vi "REPORT XLS PEDROLLO.vi"(8 "template (empty)":path, 10 "Codice":string, 11 "report file path":path) -> ()   [LabVIEW 2016]
uses:
  <vilib>/Utility/NIReport.llb/NI_report.lvclass
  <vilib>/addons/_office/NI_ReportGenerationToolkit.lvlib
  <vilib>/Utility/NIReport.llb/Excel/NI_Excel.lvclass
  <vilib>/addons/database/NI_Database_API.lvlib
  <vilib>/addons/database/_DB Variant To Data/Database Variant To Data.xnode
  <vilib>/addons/_office/excel.llb/Excel Easy Table (str).vi
  <vilib>/Utility/NIReport.llb/Append Image to Report (path wrap).vi
  <vilib>/Utility/file.llb/Read Delimited Spreadsheet (string).vi
panel:
  out "P2":dbl
  out "toll REND":dbl
  out "toll P":dbl
  out "toll H":dbl
  out "toll Q":dbl
  out "H2":dbl
  out "H1":dbl
  out "Q2":dbl
  out "Q1":dbl
  in  "template (empty) 2":path
  in  "REPORT EXCEL":bool
  out "Nomi colonne":string[](array[string])
  in  "GRAFICA":bool
  in  "exit":bool
  in  "Interpola QP2":cluster{"interpola?":bool, "order":dbl}[](array[cluster])=[{"interpola?"=FALSE, "order"=2.0}, {"interpola?"=FALSE, "order"=2.0}, {"interpola?"=FALSE, "order"=2.0}, {"interpola?"=FALSE, "order"=2.0}, {"interpola?"=FALSE, "order"=2.0}, {"interpola?"=FALSE, "order"=2.0}, {"interpola?"=FALSE, "order"=2.0}, {"interpola?"=FALSE, "order"=2.0}, {"interpola?"=FALSE, "order"=2.0}, {"interpola?"=FALSE, "order"=2.0}, {"interpola?"=FALSE, "order"=2.0}, {"interpola?"=FALSE, "order"=2.0}, {"interpola?"=FALSE, "order"=2.0}, {"interpola?"=FALSE, "order"=2.0}, {"interpola?"=FALSE, "order"=2.0}, {"interpola?"=FALSE, "order"=2.0}, {"interpola?"=FALSE, "order"=2.0}, {"interpola?"=FALSE, "order"=2.0}] caption="Interpola?"
  in  "Interpola QRpm":cluster{"interpola?":bool, "order":dbl}[](array[cluster])=[{"interpola?"=FALSE, "order"=2.0}, {"interpola?"=FALSE, "order"=2.0}, {"interpola?"=FALSE, "order"=2.0}, {"interpola?"=FALSE, "order"=2.0}, {"interpola?"=FALSE, "order"=2.0}, {"interpola?"=FALSE, "order"=2.0}, {"interpola?"=FALSE, "order"=2.0}, {"interpola?"=FALSE, "order"=2.0}, {"interpola?"=FALSE, "order"=2.0}, {"interpola?"=FALSE, "order"=2.0}, {"interpola?"=FALSE, "order"=2.0}, {"interpola?"=FALSE, "order"=2.0}, {"interpola?"=FALSE, "order"=2.0}, {"interpola?"=FALSE, "order"=2.0}, {"interpola?"=FALSE, "order"=2.0}, {"interpola?"=FALSE, "order"=2.0}, {"interpola?"=FALSE, "order"=2.0}, {"interpola?"=FALSE, "order"=2.0}] caption="Interpola?"
  in  "Interpola QH":cluster{"interpola?":bool, "order":dbl}[](array[cluster])=[{"interpola?"=FALSE, "order"=2.0}, {"interpola?"=FALSE, "order"=2.0}, {"interpola?"=FALSE, "order"=2.0}, {"interpola?"=FALSE, "order"=2.0}, {"interpola?"=FALSE, "order"=2.0}, {"interpola?"=FALSE, "order"=2.0}, {"interpola?"=FALSE, "order"=2.0}, {"interpola?"=FALSE, "order"=2.0}, {"interpola?"=FALSE, "order"=2.0}, {"interpola?"=FALSE, "order"=2.0}, {"interpola?"=FALSE, "order"=2.0}, {"interpola?"=FALSE, "order"=2.0}, {"interpola?"=FALSE, "order"=2.0}, {"interpola?"=FALSE, "order"=2.0}, {"interpola?"=FALSE, "order"=2.0}, {"interpola?"=FALSE, "order"=2.0}, {"interpola?"=FALSE, "order"=2.0}, {"interpola?"=FALSE, "order"=2.0}] caption="Interpola?"
  in  "collaudi di confronto":string[](array[string])
  in  "carica collaudi di confronto":bool
  in  "Tab Control":T1(tab)
  in  "TABELLA 3":i32(listbox)
  in  "TABELLA 2":i32(listbox)
  in  "TABELLA 1":i32(listbox)
  in  "PLOT LEGEND QH-QP2":T2(array[cluster])
  in  "PLOT LEGEND QH-QRPM":T2(array[cluster])
  out "ProvaQH-QP2":cluster{"X":dbl[], "Y":dbl[]}[](graph)
  out "ProvaQH-QRpm":cluster{"X":dbl[], "Y":dbl[]}[](graph)
  out "ProvaQH-QH":cluster{"X":dbl[], "Y":dbl[]}[](graph)
  in  "PLOT LEGEND QH-QH":T2(array[cluster])
  in  "carica collaudo in corso":bool
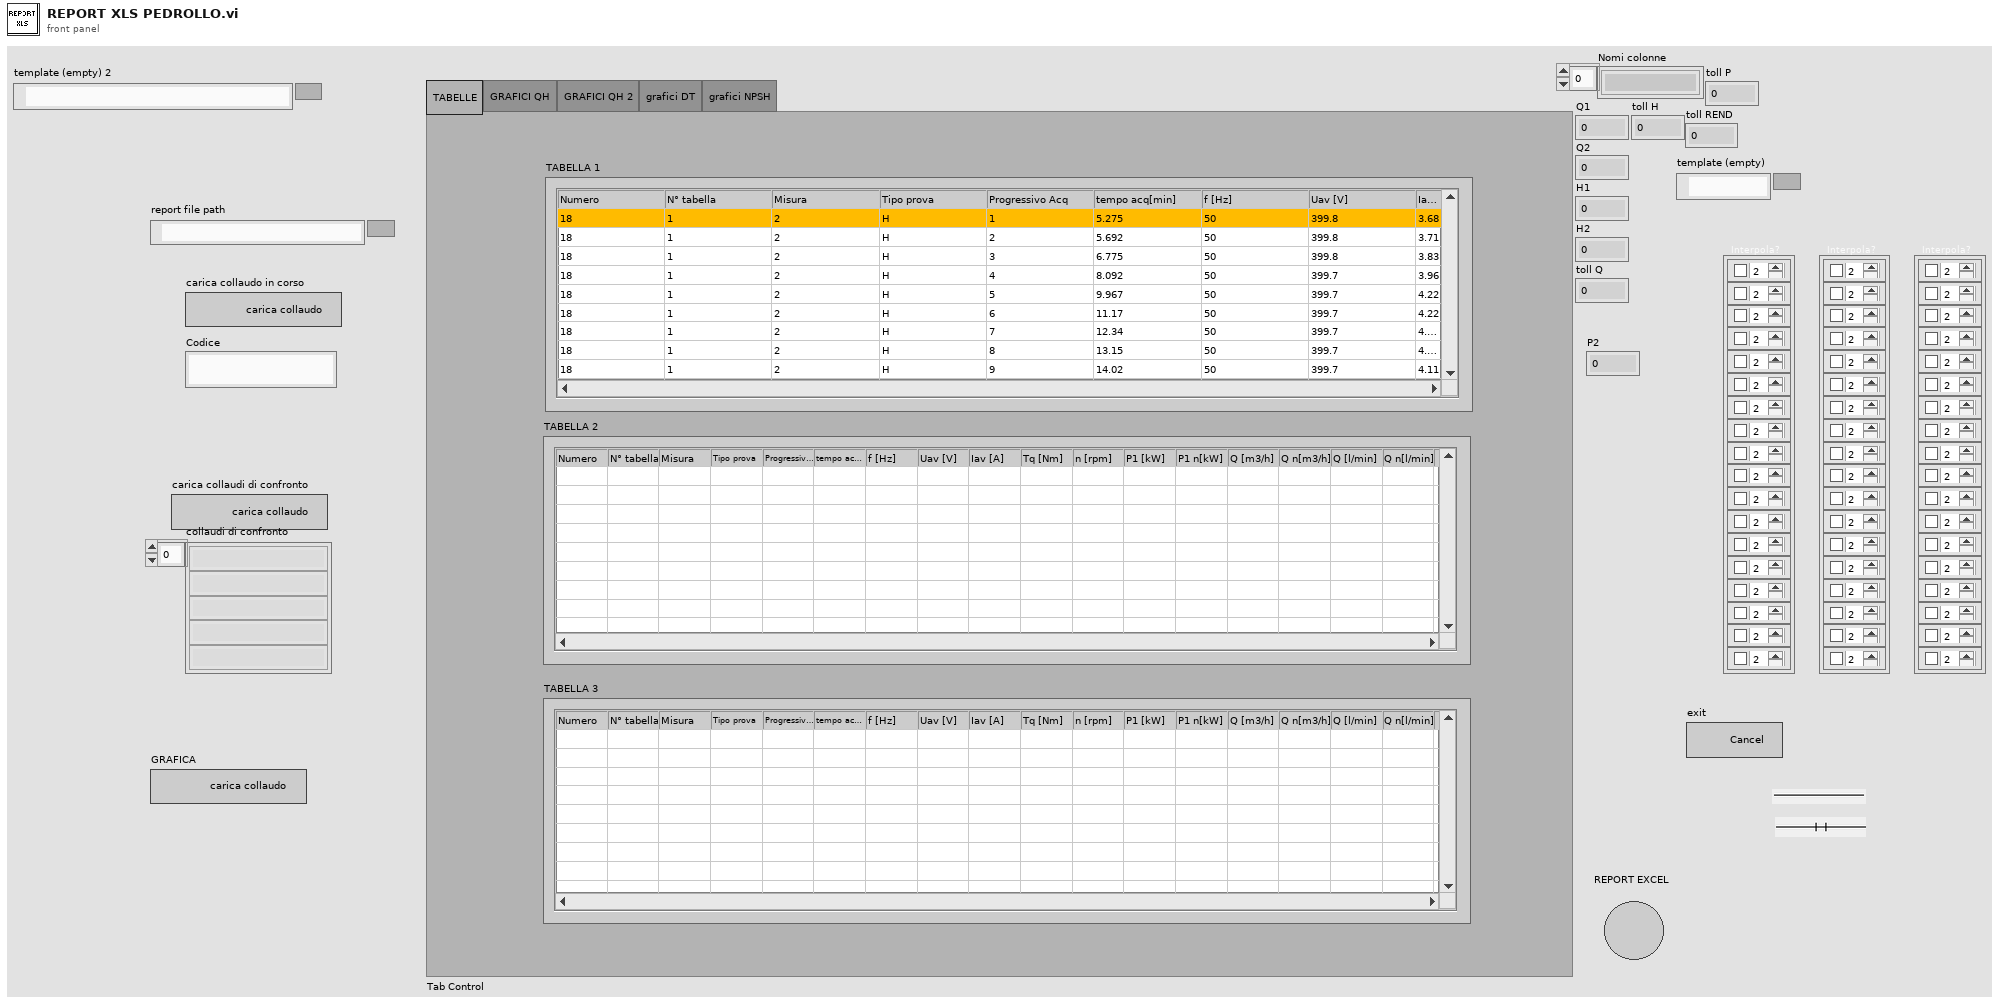
[diagram p1: front panel]
types:
  T1 = enum32{"TABELLE", "GRAFICI QH", "GRAFICI QH 2", "grafici DT", "grafici NPSH"}
  T2 = cluster{"nome plot":string, "colore":u32, "Larghezza linea":u16, "stile linea":u16, "stile punto":u16, "Visibile?":bool, "interpola?":bool, "ordine":dbl}[]
  T3 = cluster{"QH":cluster{"X":dbl[], "Y":dbl[]}[], "QRPM":cluster{"X":dbl[], "Y":dbl[]}[], "QP2":cluster{"X":dbl[], "Y":dbl[]}[]}
  T4 = enum16{"maximized", "minimized", "normal", "no change"}
  T5 = enum16{"Standard Report", "HTML", "Word", "Excel"}
  T6 = typedef "Indici.ctl" = cluster{"Q":i32, "Htot":i32, "NPSH":i32, "P3":i32, "etap":i32, "temperature":cluster{"DT":i32, "DTmarcia":i32, "DTaux":i32, "TC1":i32, "TC2":i32, "TC3":i32, "TC4":i32}, "tempo":i32, "P2":i32, "P1":i32, "etaGr":i32, "RPM":i32}
  T7 = cluster{"position (Excel)":cluster{"row":i32, "column":i32}, "name (Excel)":string, "bookmark (Word)":string}
  T8 = typedef "NI_Database_API.lvlib/Conn ObjectReference.ctl" = refnum<k1>
  T9 = typedef "Dati collaudo.ctl" = cluster{"QH freddo":T10, "QH regime":T10, "DT":T10, "NPSH":T10, "MEI":T10, "nome collaudo":string, "ResFreddo":cluster{"Curva 1":string[][]}}
  T10 = typedef "Curve prova.ctl" = cluster{"Curva 1":string[][], "Curva 2":string[][], "Curva 3":string[][]}
  T11 = cluster{"nome plot":string, "colore":u32, "Larghezza linea":u16, "stile linea":u16, "stile punto":u16, "Visibile?":bool, "interpola?":bool, "ordine":dbl}
  T12 = typedef "imagedata.ctl" = cluster{"image type":i32, "image depth":i32, "image":u8[], "mask":u8[], "colors":u32[], "Rectangle":cluster{"left":i16, "top":i16, "right":i16, "bottom":i16}}
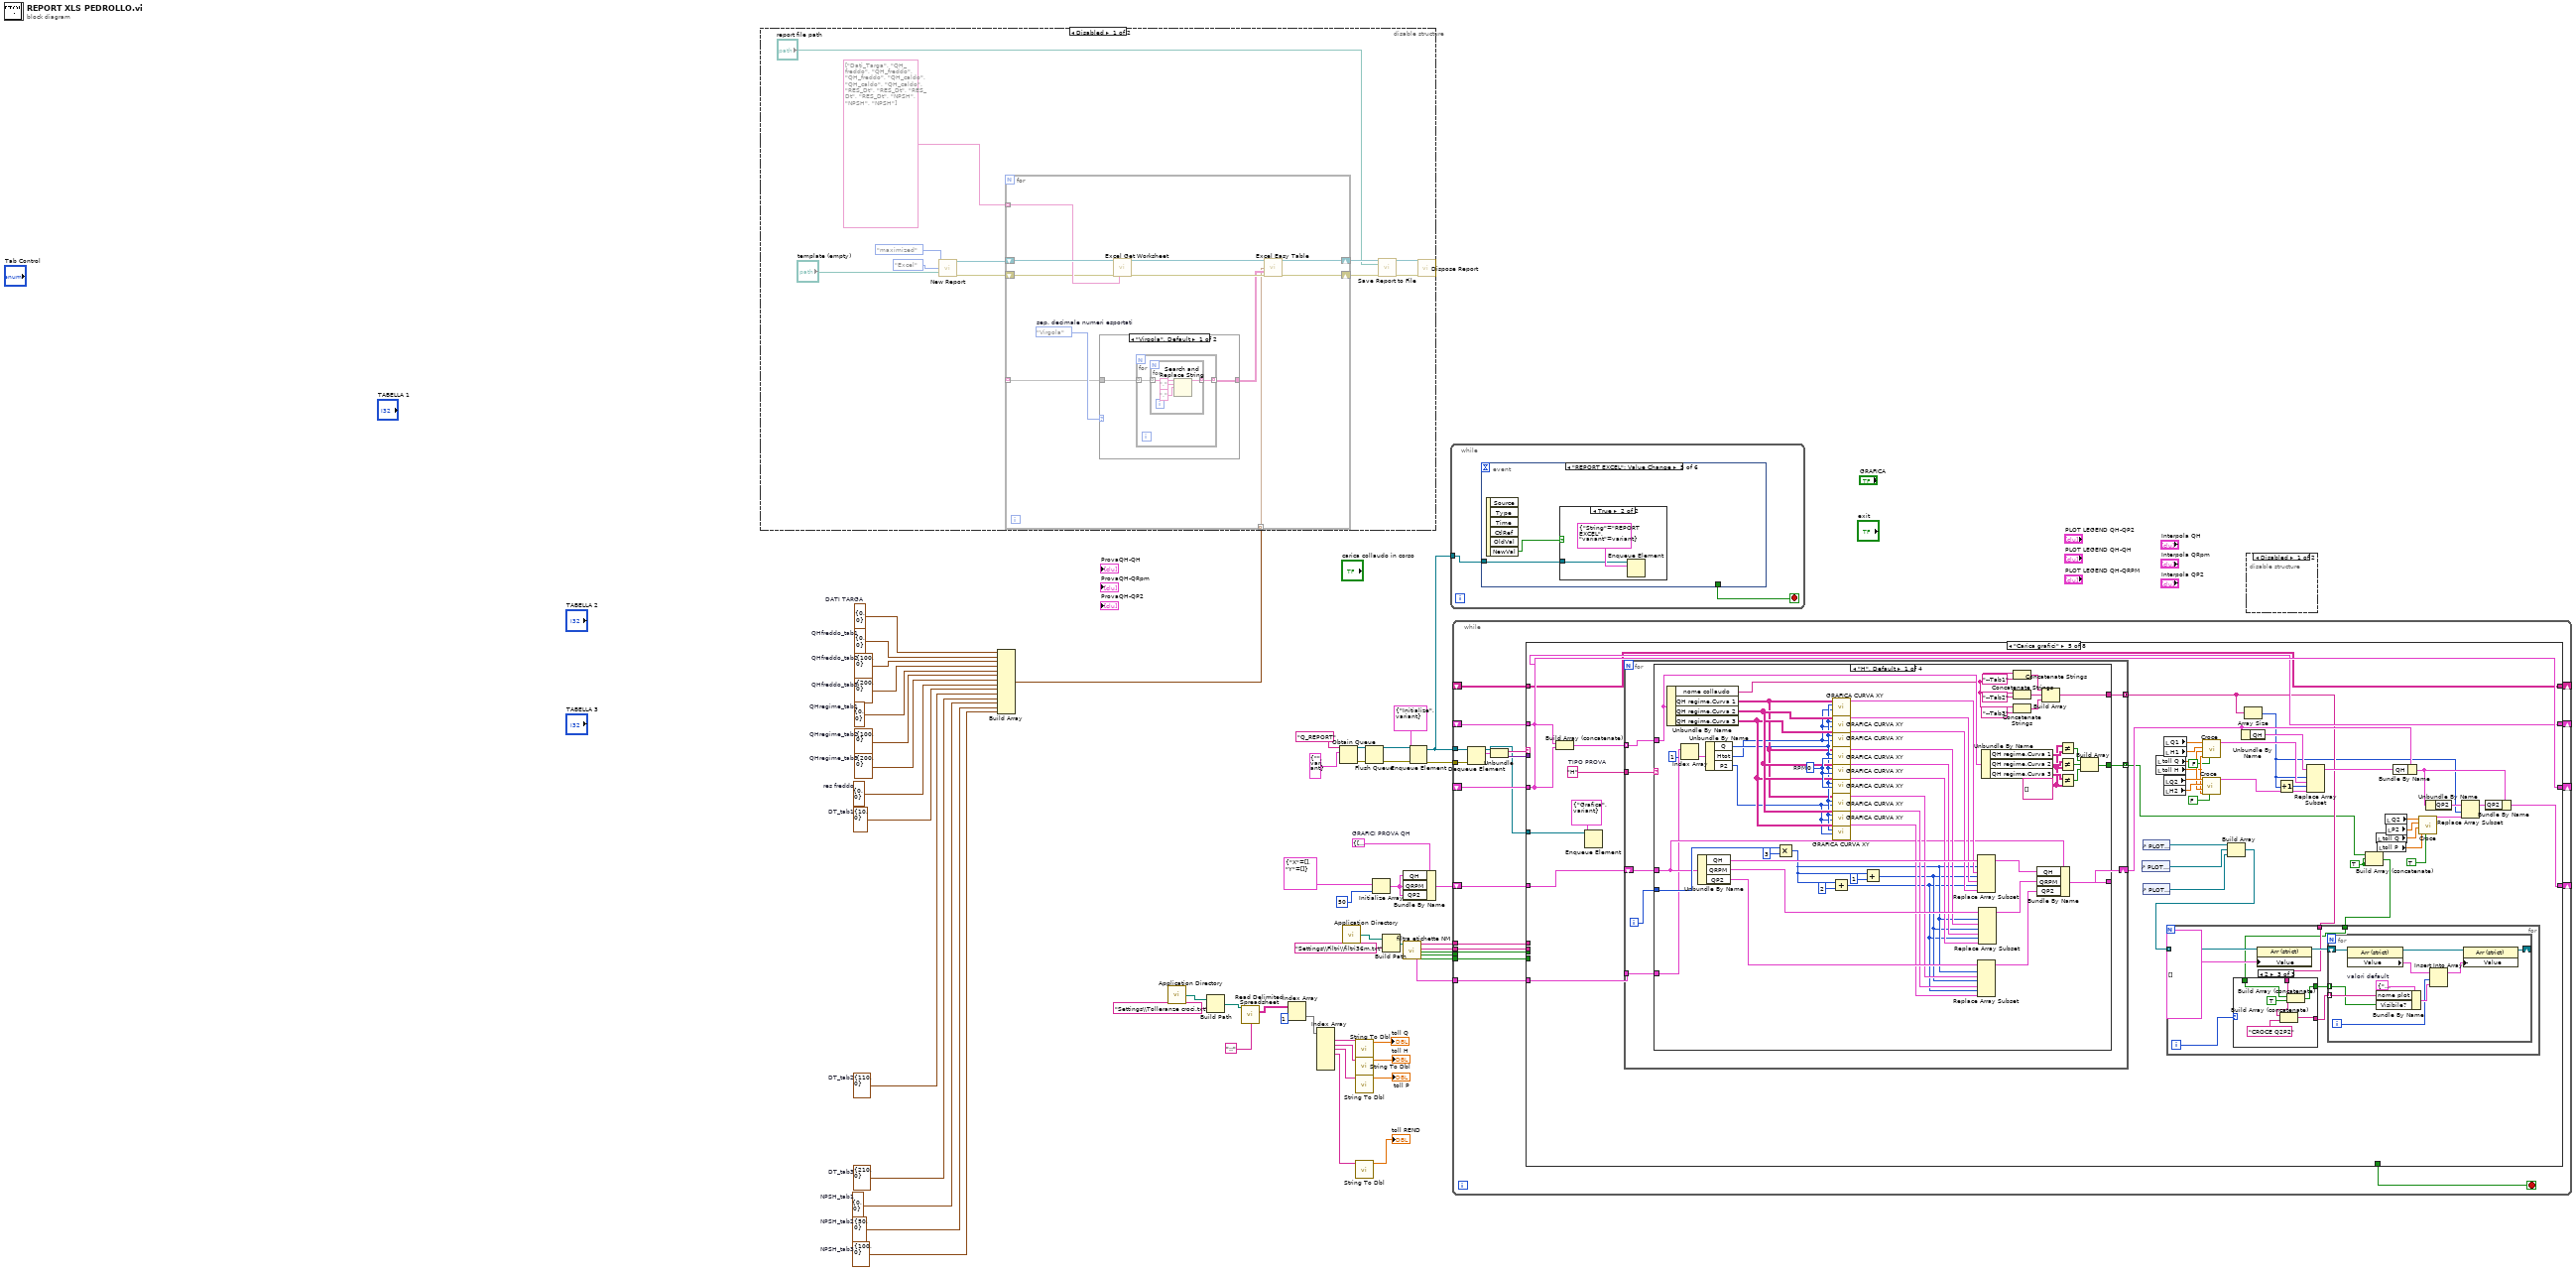
[diagram p0: block diagram]
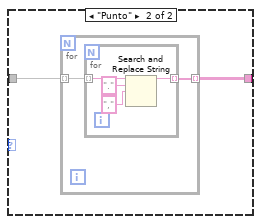
[diagram p2: hidden frame]
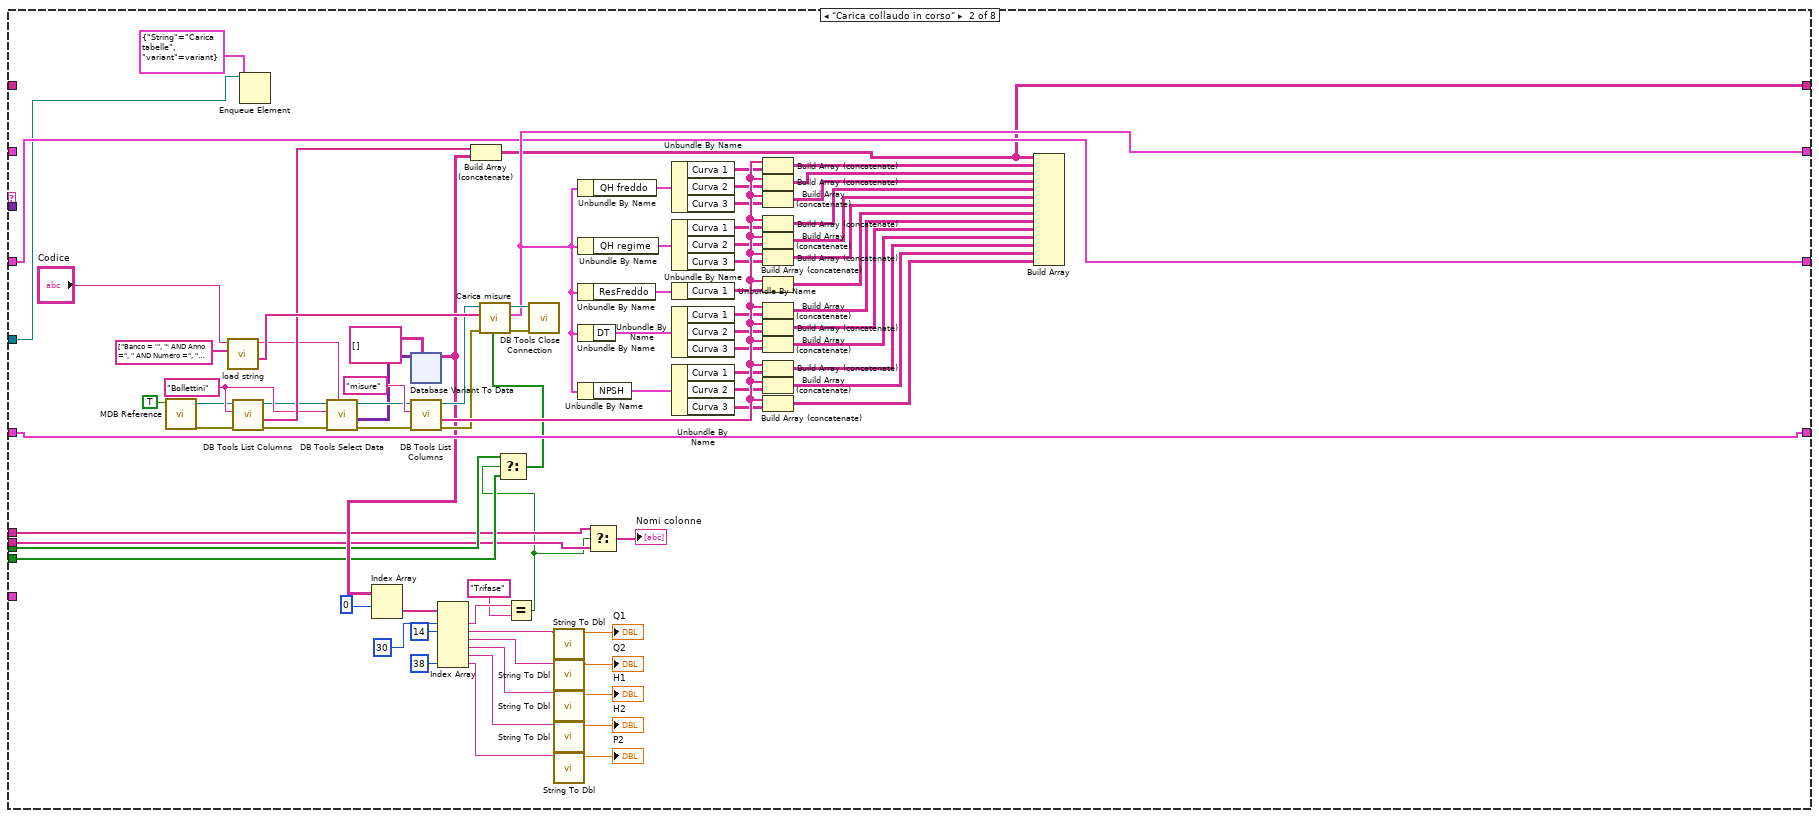
[diagram p6: hidden frame]
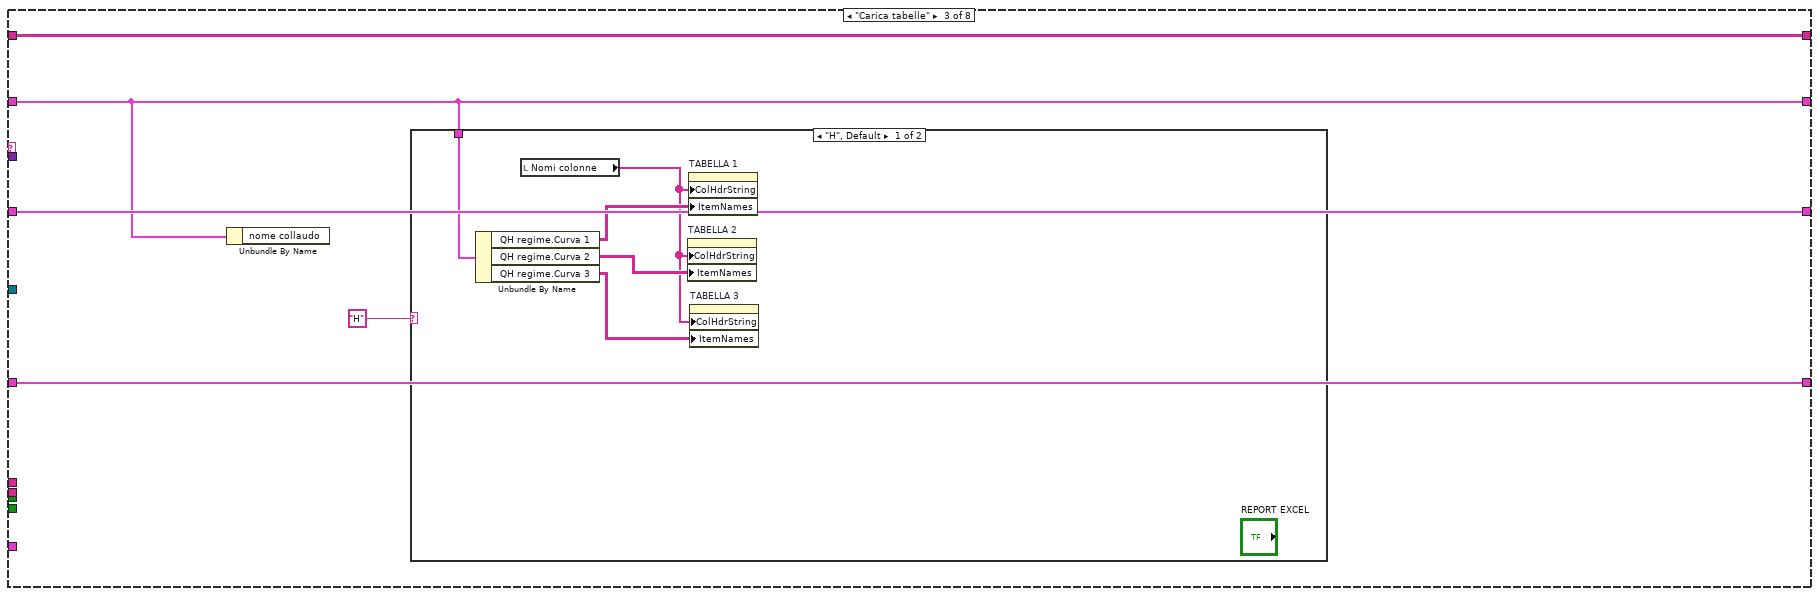
[diagram p7: hidden frame]
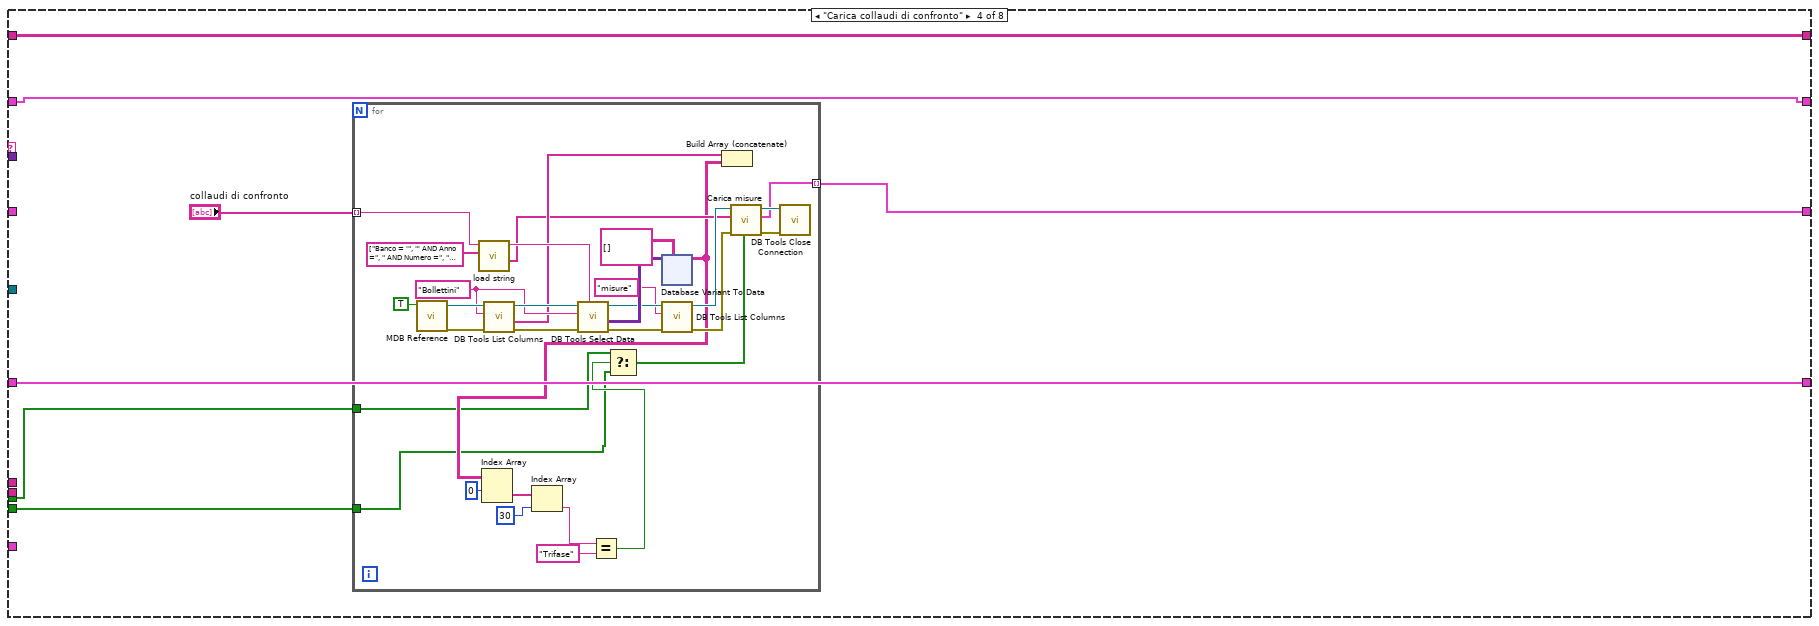
[diagram p9: hidden frame]
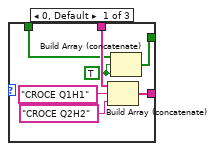
[diagram p10: hidden frame]
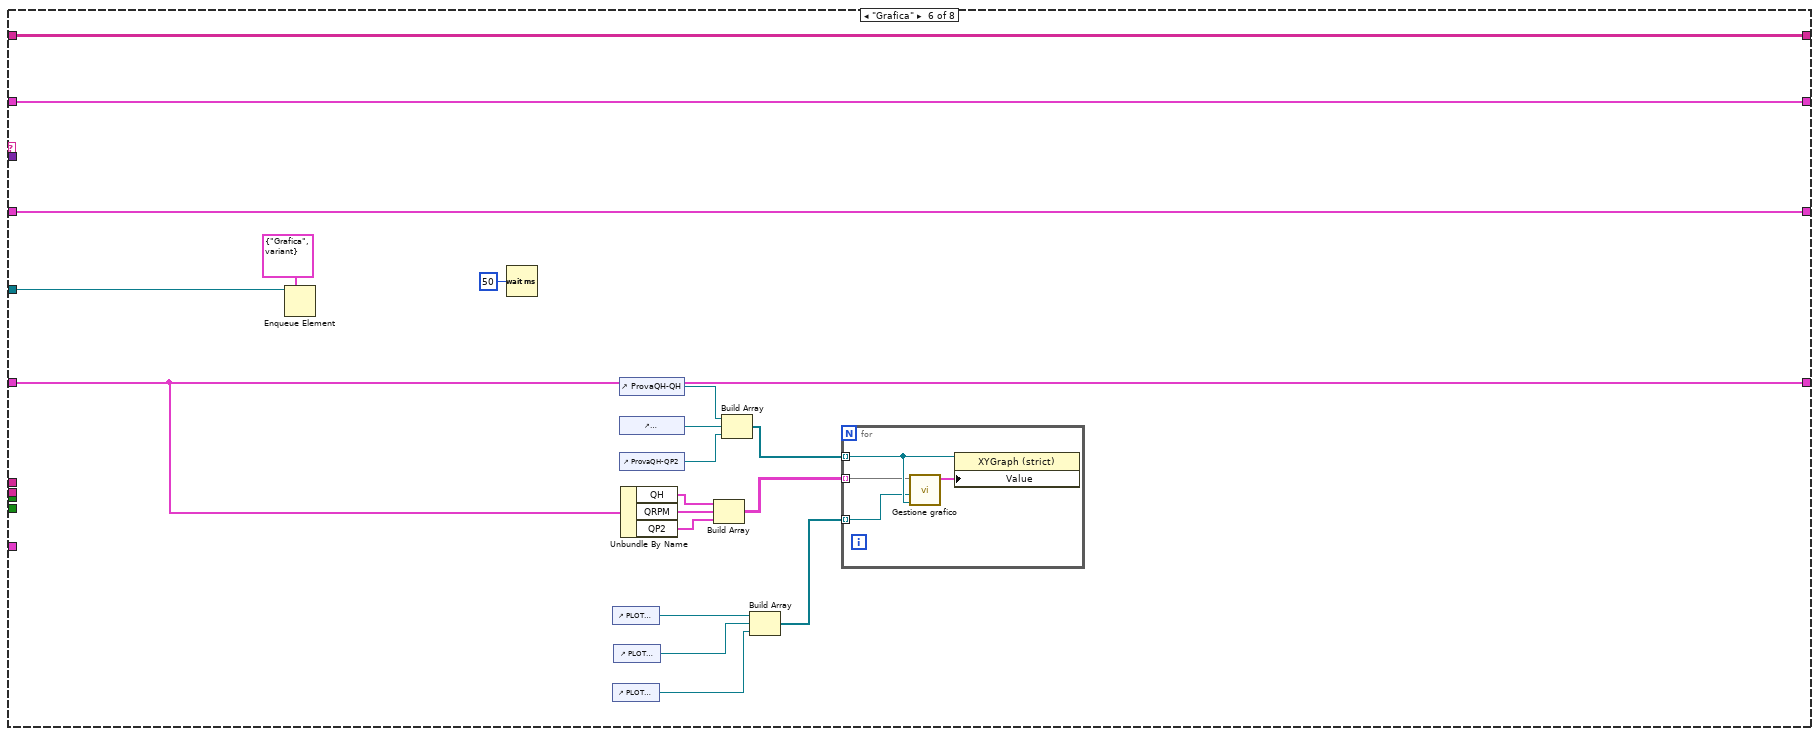
[diagram p15: hidden frame]
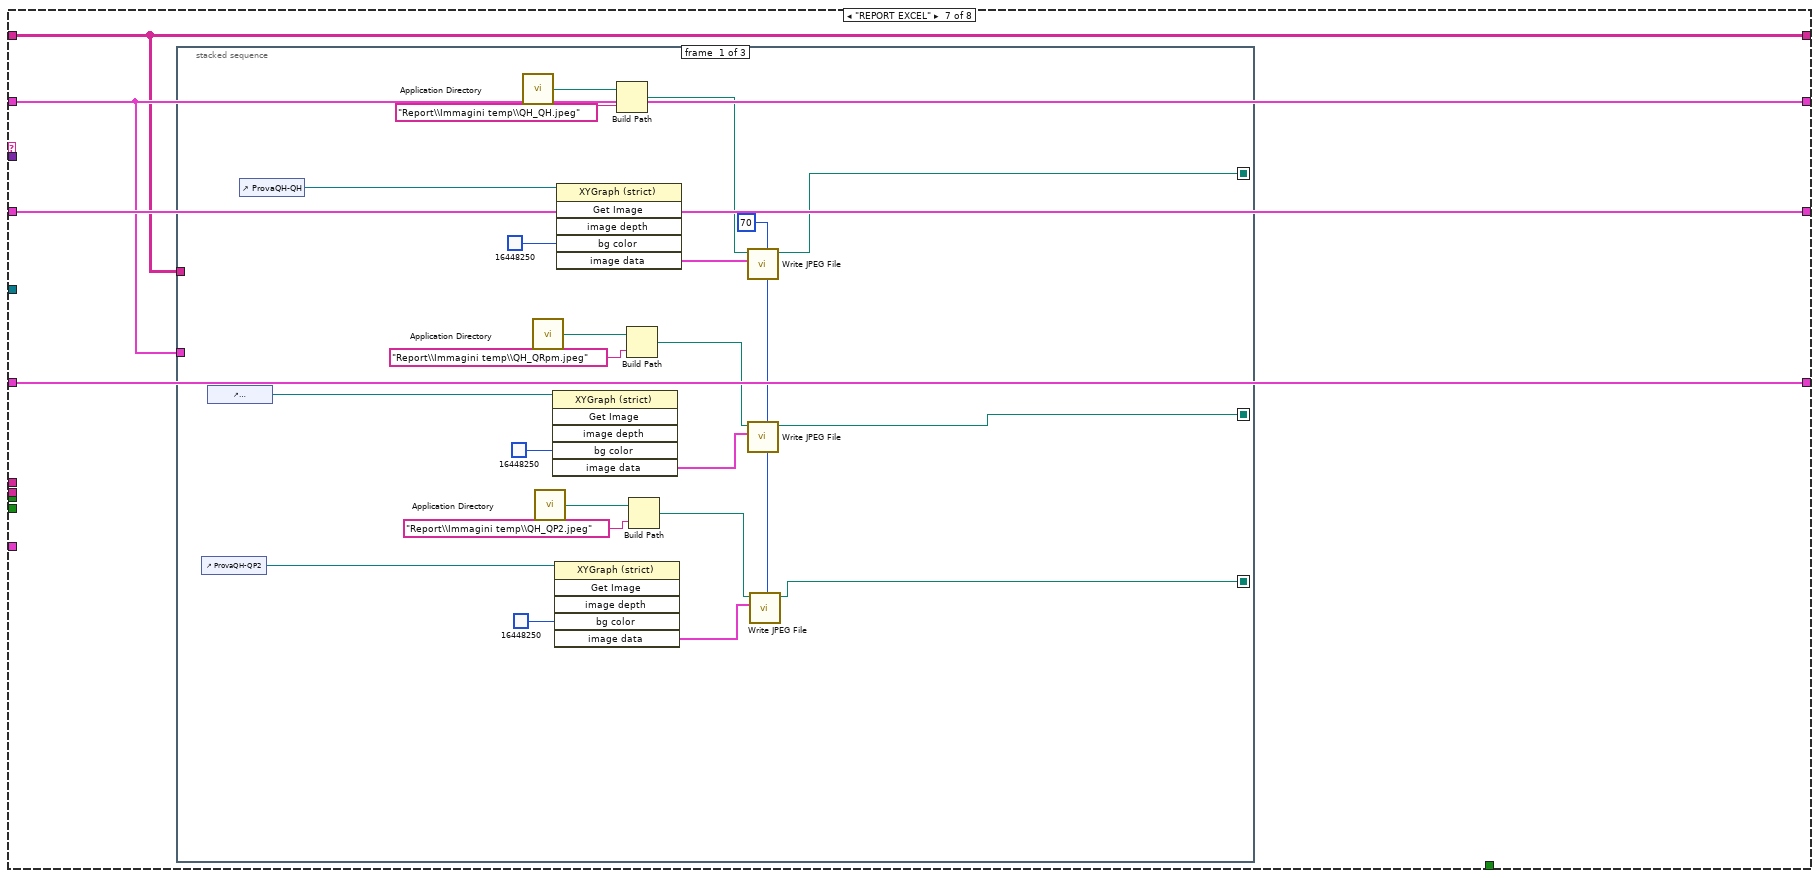
[diagram p16: hidden frame]
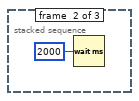
[diagram p17: hidden frame]
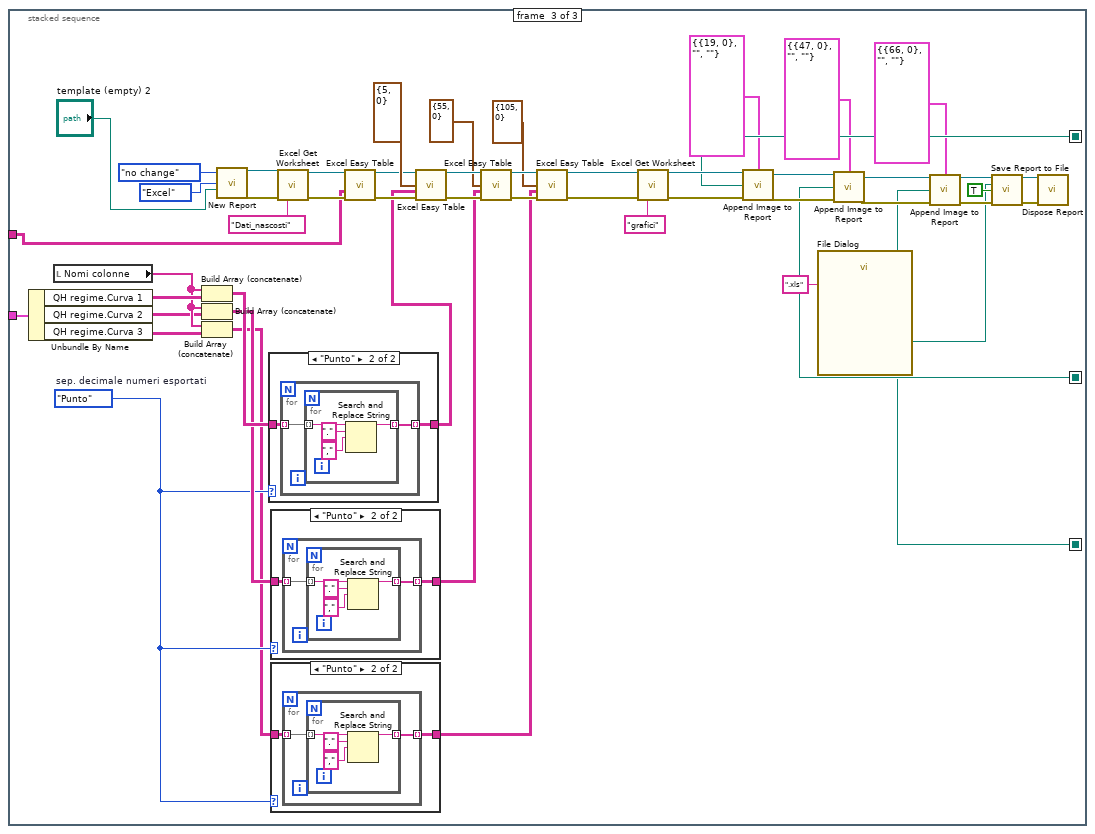
[diagram p18: hidden frame]
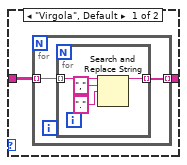
[diagram p19: hidden frame]
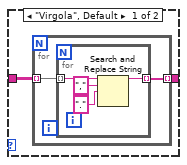
[diagram p20: hidden frame]
diagram:
  w29 = T3 {"QH"=[], "QRPM"=[], "QP2"=[]}  # GRAFICI PROVA QH
  w40 = cluster{"row":i32, "column":i32} {"row"=100, "column"=0}  # NPSH_tab3
  w41 = cluster{"row":i32, "column":i32} {"row"=50, "column"=0}  # NPSH_tab2
  w42 = cluster{"row":i32, "column":i32} {"row"=0, "column"=0}  # NPSH_tab1
  w43 = cluster{"row":i32, "column":i32} {"row"=210, "column"=0}  # DT_tab3
  w44 = cluster{"row":i32, "column":i32} {"row"=110, "column"=0}  # DT_tab2
  w45 = cluster{"row":i32, "column":i32} {"row"=10, "column"=0}  # DT_tab1
  w46 = cluster{"row":i32, "column":i32} {"row"=0, "column"=0}  # res freddo
  w47 = cluster{"row":i32, "column":i32} {"row"=200, "column"=0}  # QHregime_tab3
  w48 = cluster{"row":i32, "column":i32} {"row"=100, "column"=0}  # QHregime_tab2
  w49 = cluster{"row":i32, "column":i32} {"row"=0, "column"=0}  # QHregime_tab1
  w50 = cluster{"row":i32, "column":i32} {"row"=200, "column"=0}  # QHfreddo_tab3
  w51 = cluster{"row":i32, "column":i32} {"row"=100, "column"=0}  # QHfreddo_tab2
  w52 = cluster{"row":i32, "column":i32} {"row"=0, "column"=0}  # QHfreddo_tab1
  w53 = cluster{"row":i32, "column":i32} {"row"=0, "column"=0}  # DATI TARGA
  n1 = Build Array(w53, w52, w51, w50, w49, w48, w47, w46, w45, w44, w43, w42, w41, w40) -> (w39:cluster{"row":i32, "column":i32}[])
  n2 = disable-structure shown="Disabled" {
    disable-tunnel: w39 -> [w59 _]
    frame Disabled {
      n3 = call <vilib>:"New Report.vi"("window state (normal)"=T4."maximized", "report type"=T5."Excel", "template (empty)"="template (empty)") -> ("report out"=w63:refnum<class "NI_report.lvclass">, "error out"=w61:errorcluster)  [unwired: 11 in]
      n4 = for {
        shift-right: [w76] -> w56
        shift-left: w63 -> [w75]
        tunnel: string[] ["Dati_Targa", "QH_freddo", "QH_freddo", "QH_freddo", "QH_caldo", "QH_caldo", "QH_caldo", "RES_Dt", "RES_Dt", "RES_Dt", "RES_Dt", "NPSH", "NPSH", "NPSH"] -> [w73] mode=indexing
        shift-right: [w70] -> w58
        shift-left: w61 -> [w72]
        tunnel: _ -> [w68] mode=indexing
        tunnel: w59 -> [w66] mode=indexing
        w69 = enum16{"Virgola", "Punto"}."Virgola"  # sep. decimale numeri esportati
        n5 = case shown="\"Virgola\", Default" w69 {
          tunnel: w68 -> [w78 w86]
          tunnel: [w77 w85] -> w67
          frame "Virgola", Default {
            n6 = for {
              tunnel: w78 -> [w80] mode=indexing
              tunnel: [w79] -> w77 mode=indexing
              n7 = for {
                tunnel: w80 -> [w84] mode=indexing
                tunnel: [w81] -> w79 mode=indexing
                n8 = Search and Replace String(input string=w84, search string=",", replace string="." ("search string")) -> (result string=w81:string)  [unwired: 5 in, 3 out]
              }
            }
          }
          frame "Punto" {
            n9 = for {
              tunnel: w86 -> [w88] mode=indexing
              tunnel: [w87] -> w85 mode=indexing
              n10 = for {
                tunnel: w88 -> [w92] mode=indexing
                tunnel: [w89] -> w87 mode=indexing
                n11 = Search and Replace String(input string=w92, search string=".", replace string="," ("search string")) -> (result string=w89:string)  [unwired: 5 in, 3 out]
              }
            }
          }
        }
        n12 = call <vilib>:"Excel Get Worksheet.vi"("report in"=w75, "error in (no error)"=w72, "name (\"\")"=w73) -> ("report out"=w74:refnum<class "NI_report.lvclass">, "error out"=w71:errorcluster)  [unwired: 11 in]
        n13 = call-poly <vilib>:"Excel Easy Table.vi"("report in"=w74, "start (0, 0)"=w66, "text data"=w67, "error in (no error)"=w71) -> ("report out"=w76:refnum<class "NI_report.lvclass">, "error out"=w70:errorcluster)  [unwired: 7 in, 3 out]
      }
      n14 = call-dynamic "Save Report to File.vi"("report in"=w56, "report file path"="report file path", "error in (no error)"=w58) -> ("report out"=w55:refnum<class "NI_report.lvclass">, "error out"=w57:errorcluster)  [unwired: 11 in]
      n15 = call-dynamic "Dispose Report.vi"("report in"=w55, "error in (no error)"=w57) -> ()  [unwired: 13 in, 1 out]
    }
    frame Enabled {
    }
  }
  n16 = call <vilib>:"Application Directory.vi"() -> ("Application Directory"=w15:path)
  n17 = Build Path(base path=w15, name or relative path="Settings\\Tolleranze croci.txt") -> (appended path=w13:path)
  n18 = call-poly <vilib>:"Read Delimited Spreadsheet.vi"("file path (dialog if empty)"=w13, "delimiter (\\t)"="::" ("delimiter (\\t)")) -> ("all rows"=w11:string[][])  [unwired: 8 in, 5 out]
  n19 = Index Array(array=w11, index (col)=1 ("disabled index (col)")) -> (element=w9:string[])  [unwired: 1 in]
  n20 = Index Array(array=w9) -> (element #1=w8:string, element #2=w6:string, element #3=w5:string, element #4=w4:string)  [unwired: 7 in, 3 out]
  n21 = Obtain Queue(name (unnamed)="Q_REPORT", element data type=cluster{"String":string, "variant":variant} {"String"="", "variant"=variant} ("element")) -> (queue out=w35:refnum<queue>, error out=w36:errorcluster)  [unwired: 3 in, 1 out]
  n22 = call <vilib>:"Application Directory.vi"() -> ("Application Directory"=w22:path)
  n23 = call "String To Dbl.vi"("String"=w8) -> ("Numeric"=→"toll Q":dbl)  [unwired: 10 in]
  n24 = call "String To Dbl.vi"("String"=w6) -> ("Numeric"=→"toll H":dbl)  [unwired: 10 in]
  n25 = call "String To Dbl.vi"("String"=w5) -> ("Numeric"=→"toll P":dbl)  [unwired: 10 in]
  n26 = call "String To Dbl.vi"("String"=w4) -> ("Numeric"=→"toll REND":dbl)  [unwired: 10 in]
  n27 = Flush Queue(queue=w35, error in (no error)=w36) -> (queue out=w37:refnum<queue>, error out=w38:errorcluster)  [unwired: 1 out]
  n28 = Initialize Array(cluster{"X":dbl[], "Y":dbl[]} {"X"=[], "Y"=[]} ("QP"), 50 ("dimension size")) -> (w25:cluster{"X":dbl[], "Y":dbl[]}[])
  n29 = Build Path(base path=w22, name or relative path="Settings\\Filtri\\filtri36m.txt") -> (appended path=w24:path)
  n30 = Bundle By Name(cluster=w29, "QH"=w25, "QRPM"=w25, "QP2"=w25) -> (w28:T3)
  n31 = call "filtra etichette NM.vi"("File filtri path"=w24) -> ("indici grafici m,3,6"=w21:T6[], "Array 3ph3ch"=w17:string[], "Array 1ph"=w16:string[], "Filtro 3ph3ch"=w20:bool[], "Filtro 3ph6ch"=w19:bool[], "Filtro 1ph"=w18:bool[])  [unwired: 11 in, 2 out]
  n32 = Enqueue Element(queue=w37, element=cluster{"String":string, "variant":variant} {"String"="Initialize", "variant"=variant}, error in (no error)=w38) -> (queue out=w30:refnum<queue>, error out=w33:errorcluster)  [unwired: 1 in, 1 out]
  n33 = while {
    tunnel: w30 -> [w94]
    stop <- w93 stop-if-true
    n34 = event shown="[4] \"REPORT EXCEL\": Value Change" {
      selector: _ -> [_ _ _ _ _ _]
      dyn-events: _ -> [_ _ _ _ _ _]
      timeout: _ -> [_ _ _ _ _ _]
      tunnel: w94 -> [_ w95 w97 w99 w102 _]
      tunnel: [_ _ _ _ _ TRUE] -> w93
      event Timeout {
        n35 = event-data() -> ()  [unwired: 1 in, 3 out]
      }
      event "carica collaudo in corso": Value Change {
        n36 = event-data() -> ()  [unwired: 1 in, 6 out]
        n37 = Enqueue Element(queue=w95, element=cluster{"String":string, "variant":variant} {"String"="Carica collaudo in corso", "variant"=variant}) -> ()  [unwired: 2 in, 3 out]
      }
      event "carica collaudi di confronto": Value Change {
        n38 = event-data() -> ()  [unwired: 1 in, 6 out]
        n39 = Enqueue Element(queue=w97, element=cluster{"String":string, "variant":variant} {"String"="Carica collaudi di confronto", "variant"=variant}) -> ()  [unwired: 2 in, 3 out]
      }
      event "GRAFICA": Value Change {
        n40 = event-data() -> ()  [unwired: 1 in, 6 out]
        n41 = Enqueue Element(queue=w99, element=cluster{"String":string, "variant":variant} {"String"="Carica grafici", "variant"=variant}) -> ()  [unwired: 2 in, 3 out]
      }
      event "REPORT EXCEL": Value Change {
        n42 = event-data() -> ("NewVal"=w101:bool)  [unwired: 1 in, 5 out]
        n43 = case shown="True" w101 {
          tunnel: w102 -> [_ w103]
          frame False {
          }
          frame True {
            n44 = Enqueue Element(queue=w103, element=cluster{"String":string, "variant":variant} {"String"="REPORT EXCEL", "variant"=variant}) -> ()  [unwired: 2 in, 3 out]
          }
        }
      }
      event "exit": Value Change {
        n45 = event-data() -> ()  [unwired: 1 in, 6 out]
      }
    }
  }
  n46 = while {
    tunnel: w30 -> [w125]
    tunnel: w33 -> [w124]
    shift-right: [w119] -> _
    shift-left: _ -> [w118]
    shift-right: [w117] -> _
    shift-left: _ -> [w116]
    shift-right: [w115] -> _
    shift-left: _ -> [w114]
    shift-right: [w112] -> _
    shift-left: w28 -> [w113]
    tunnel: w21 -> [w111]
    tunnel: w20 -> [w109]
    tunnel: w19 -> [_]
    tunnel: w18 -> [w110]
    tunnel: w17 -> [w107]
    tunnel: w16 -> [w106]
    stop <- w121 stop-if-true
    n47 = Dequeue Element(queue=w125, error in (no error)=w124) -> (queue out=w108:refnum<queue>, element=w123:cluster{"String":string, "variant":variant})  [unwired: 1 in, 2 out]
    n48 = Unbundle(w123) -> ("String"=w122:string, "variant"=w120:variant)
    n49 = case shown="\"Carica grafici\"" w122 {
      tunnel: [_ _ _ _ _ _ _ TRUE] -> w121
      tunnel: w120 -> [_ _ _ _ _ _ _ _]
      tunnel: [w126 w142 w261 w269 w385 w501 w506 w636] -> w119
      tunnel: w118 -> [w126 _ w261 w269 w385 w501 w506 w636]
      tunnel: [w128 w158 w260 w272 w390 w500 w509 w634] -> w117
      tunnel: w116 -> [w128 w158 w260 _ w390 w500 w509 w634]
      tunnel: [w127 w160 w257 w270 w389 w499 w507 w635] -> w115
      tunnel: w114 -> [w127 _ w257 w270 w389 w499 w507 w635]
      tunnel: w113 -> [w129 w159 w259 w271 w386 w487 w508 w633]
      tunnel: [w129 w159 w259 w271 w361 w487 w508 w633] -> w112
      tunnel: w111 -> [_ _ _ _ w384 _ _ _]
      tunnel: w110 -> [_ w151 _ w268 _ _ _ _]
      tunnel: w109 -> [_ w150 _ w267 _ _ _ _]
      tunnel: w108 -> [_ w147 _ _ w382 w485 _ _]
      tunnel: w107 -> [_ w146 _ _ _ _ _ _]
      tunnel: w106 -> [_ w145 _ _ _ _ _ _]
      frame "Initialize", Default {
      }
      frame "Carica collaudo in corso" {
        w204 = "Bollettini" ("table")
        n50 = call "MDB Reference.vi"("Collaudi T/motori F"=TRUE ("NM?")) -> ("error out"=w202:errorcluster, "Refnum out"=w200:T8)  [unwired: 8 in, 1 out]
        n51 = call "load string.vi"("Array in"=string[] ["Banco = '", "' AND Anno =", " AND Numero =", " And Tipo_Prova='", "'"], "Codice"="Codice") -> ("ID bollettino"=w212:string[], "String command"=w198:string)  [unwired: 7 in, 1 out]
        n52 = call <vilib>:"DB Tools List Columns.vi"("error in (no error)"=w202, "table"=w204, "connection reference"=w200) -> ("error out"=w203:errorcluster, "columns"=w205:string[], "connection reference out"=w201:T8)  [unwired: 1 in, 1 out]
        n53 = Enqueue Element(queue=w147, element=cluster{"String":string, "variant":variant} {"String"="Carica tabelle", "variant"=variant}) -> ()  [unwired: 2 in, 3 out]
        n54 = call <vilib>:"DB Tools Select Data.vi"("condition"=w198, "error in (no error)"=w203, "table"=w204, "connection reference"=w201) -> ("error out"=w206:errorcluster, "data"=w196:variant[][], "connection reference out"=w208:T8)  [unwired: 2 in]
        n55 = xnode "Database Variant To Data"("database variant"=w196, "type"=string[][] [] ("Item Names")) -> ("data"=w152:string[][])  [unwired: 1 in, 1 out]
        n56 = Index Array(array=w152, index (row)=0 ("disabled index (col)")) -> (element=w156:string[])  [unwired: 1 in]
        n57 = call <vilib>:"DB Tools List Columns.vi"("error in (no error)"=w206, "table"="misure", "connection reference"=w208) -> ("error out"=w207:errorcluster, "columns"=w211:string[], "connection reference out"=w209:T8)  [unwired: 1 in, 1 out]
        n58 = Index Array(array=w156, index #1=30 ("index"), index #2=14 ("index"), index #6=38 ("index")) -> (element #1=w154:string, element #2=w139:string, element #3=w137:string, element #4=w136:string, element #5=w135:string, element #6=w134:string)  [unwired: 3 in]
        n59 = Build Array (concatenate)(w205, w152) -> (w142:string[][])
        n60 = Equal?(x=w154, y="Trifase") -> (x = y?=w143:bool)
        n61 = Select(t=w150, s=w143, f=w151) -> (s? t:f=w149:bool[])
        n62 = call "Carica misure.vi"("Filtro 3ph6ch"=w149, "error in (no error)"=w207, "ID bollettino"=w212, "Refnum in"=w209) -> ("error out"=w194:errorcluster, "Dati prove out"=w160:T9, "Refnum out"=w193:T8)  [unwired: 5 in]
        n63 = call <vilib>:"DB Tools Close Connection.vi"("error in (no error)"=w194, "connection reference"=w193) -> ()  [unwired: 5 in, 1 out]
        n64 = call "String To Dbl.vi"("String"=w139) -> ("Numeric"=→"Q1":dbl)  [unwired: 10 in]
        n65 = call "String To Dbl.vi"("String"=w137) -> ("Numeric"=→"Q2":dbl)  [unwired: 10 in]
        n66 = call "String To Dbl.vi"("String"=w136) -> ("Numeric"=→"H1":dbl)  [unwired: 10 in]
        n67 = call "String To Dbl.vi"("String"=w135) -> ("Numeric"=→"H2":dbl)  [unwired: 10 in]
        n68 = call "String To Dbl.vi"("String"=w134) -> ("Numeric"=→"P2":dbl)  [unwired: 10 in]
        n69 = Unbundle By Name(w160) -> ("QH freddo"=w161:T10)
        n70 = Unbundle By Name(w160) -> ("QH regime"=w162:T10)
        n71 = Unbundle By Name(w160) -> ("ResFreddo"=w164:cluster{"Curva 1":string[][]})
        n72 = Unbundle By Name(w160) -> ("DT"=w163:T10)
        n73 = Unbundle By Name(w160) -> ("NPSH"=w165:T10)
        n74 = Select(t=w146, s=w143, f=w145) -> (s? t:f=→"Nomi colonne":string[])
        n75 = Unbundle By Name(w161) -> ("Curva 1"=w166:string[][], "Curva 2"=w167:string[][], "Curva 3"=w168:string[][])
        n76 = Unbundle By Name(w162) -> ("Curva 1"=w172:string[][], "Curva 2"=w173:string[][], "Curva 3"=w174:string[][])
        n77 = Unbundle By Name(w164) -> ("Curva 1"=w178:string[][])
        n78 = Unbundle By Name(w163) -> ("Curva 1"=w179:string[][], "Curva 2"=w180:string[][], "Curva 3"=w181:string[][])
        n79 = Unbundle By Name(w165) -> ("Curva 1"=w186:string[][], "Curva 2"=w187:string[][], "Curva 3"=w188:string[][])
        n80 = Build Array (concatenate)(w211, w166) -> (w169:string[][])
        n81 = Build Array (concatenate)(w211, w167) -> (w170:string[][])
        n82 = Build Array (concatenate)(w211, w168) -> (w171:string[][])
        n83 = Build Array (concatenate)(w211, w172) -> (w175:string[][])
        n84 = Build Array (concatenate)(w211, w173) -> (w176:string[][])
        n85 = Build Array (concatenate)(w211, w174) -> (w177:string[][])
        n86 = Build Array (concatenate)(w211, w178) -> (w182:string[][])
        n87 = Build Array (concatenate)(w211, w179) -> (w183:string[][])
        n88 = Build Array (concatenate)(w211, w180) -> (w184:string[][])
        n89 = Build Array (concatenate)(w211, w181) -> (w185:string[][])
        n90 = Build Array (concatenate)(w211, w186) -> (w189:string[][])
        n91 = Build Array (concatenate)(w211, w187) -> (w190:string[][])
        n92 = Build Array (concatenate)(w211, w188) -> (w191:string[][])
        n93 = Build Array(w142, w169, w170, w171, w175, w176, w177, w182, w183, w184, w185, w189, w190, w191) -> ()  [unwired: 1 out]
      }
      frame "Carica tabelle" {
        n94 = Unbundle By Name(w257) -> ()  [unwired: 1 out]
        n95 = case shown="\"H\", Default" "H" {
          tunnel: w257 -> [w266 _]
          frame "H", Default {
            n96 = Unbundle By Name(w266) -> ("QH regime.Curva 1"=w265:string[][], "QH regime.Curva 2"=w264:string[][], "QH regime.Curva 3"=w263:string[][])
            n97 = local read "Nomi colonne"() -> (w262:string[])
            n98 = property on="TABELLA 2" class="MCListbox (strict)"("ColHdrString"=w262, "ItemNames"=w264) -> ()  [unwired: 2 in, 2 out]
            n99 = property on="TABELLA 1" class="MCListbox (strict)"("ColHdrString"=w262, "ItemNames"=w265) -> ()  [unwired: 2 in, 2 out]
            n100 = property on="TABELLA 3" class="MCListbox (strict)"("ColHdrString"=w262, "ItemNames"=w263) -> ()  [unwired: 2 in, 2 out]
          }
          frame "True" {
          }
        }
      }
      frame "Carica collaudi di confronto" {
        n101 = for {
          tunnel: "collaudi di confronto" -> [w285] mode=indexing
          tunnel: [w284] -> w272 mode=indexing
          tunnel: w268 -> [w276]
          tunnel: w267 -> [w275]
          w293 = "Bollettini" ("table")
          n102 = call "MDB Reference.vi"("Collaudi T/motori F"=TRUE ("NM?")) -> ("error out"=w295:errorcluster, "Refnum out"=w297:T8)  [unwired: 8 in, 1 out]
          n103 = call "load string.vi"("Array in"=string[] ["Banco = '", "' AND Anno =", " AND Numero =", " And Tipo_Prova='", "'"], "Codice"=w285) -> ("ID bollettino"=w286:string[], "String command"=w298:string)  [unwired: 7 in, 1 out]
          n104 = call <vilib>:"DB Tools List Columns.vi"("error in (no error)"=w295, "table"=w293, "connection reference"=w297) -> ("error out"=w294:errorcluster, "columns"=w292:string[], "connection reference out"=w296:T8)  [unwired: 1 in, 1 out]
          n105 = call <vilib>:"DB Tools Select Data.vi"("condition"=w298, "error in (no error)"=w294, "table"=w293, "connection reference"=w296) -> ("error out"=w291:errorcluster, "data"=w300:variant[][], "connection reference out"=w289:T8)  [unwired: 2 in]
          n106 = xnode "Database Variant To Data"("database variant"=w300, "type"=string[][] [] ("Item Names")) -> ("data"=w277:string[][])  [unwired: 1 in, 1 out]
          n107 = Index Array(array=w277, index (row)=0 ("disabled index (col)")) -> (element=w281:string[])  [unwired: 1 in]
          n108 = Index Array(array=w281, index=30) -> (element=w283:string)
          n109 = Equal?(x=w283, y="Trifase") -> (x = y?=w278:bool)
          n110 = Select(t=w275, s=w278, f=w276) -> (s? t:f=w274:bool[])
          n111 = call <vilib>:"DB Tools List Columns.vi"("error in (no error)"=w291, "table"="misure", "connection reference"=w289) -> ("error out"=w290:errorcluster, "connection reference out"=w288:T8)  [unwired: 1 in, 2 out]
          n112 = Build Array (concatenate)(w292, w277) -> ()  [unwired: 1 out]
          n113 = call "Carica misure.vi"("Filtro 3ph6ch"=w274, "error in (no error)"=w290, "ID bollettino"=w286, "Refnum in"=w288) -> ("error out"=w302:errorcluster, "Dati prove out"=w284:T9, "Refnum out"=w303:T8)  [unwired: 5 in]
          n114 = call <vilib>:"DB Tools Close Connection.vi"("error in (no error)"=w302, "connection reference"=w303) -> ()  [unwired: 5 in, 1 out]
        }
      }
      frame "Carica grafici" {
        w365 = TRUE
        w387 = "H"  # TIPO PROVA
        n115 = Build Array (concatenate)(w389, w390) -> (w388:T9[])
        n116 = Enqueue Element(queue=w382, element=cluster{"String":string, "variant":variant} {"String"="Grafica", "variant"=variant}) -> ()  [unwired: 2 in, 3 out]
        n117 = for {
          tunnel: w388 -> [w430] mode=indexing
          tunnel: w387 -> [w431]
          shift-right: [w427] -> w366
          shift-left: w386 -> [w429]
          tunnel: [w426] -> w363 mode=concatenating
          tunnel: w384 -> [w425]
          tunnel: [w424] -> w362 mode=concatenating
          i -> [w428]
          n118 = case shown="\"H\", Default" w431 {
            tunnel: w430 -> [w444 _ _ _]
            tunnel: w429 -> [w460 _ _ _]
            tunnel: w428 -> [w480 _ _ _]
            tunnel: [w453 _ _ _] -> w427
            tunnel: [w452 _ _ _] -> w426
            tunnel: w425 -> [w451 _ _ _]
            tunnel: [w436 _ _ _] -> w424
            frame "H", Default {
              w440 = string[][] [] ("y")
              w471 = 0  # RPM
              n119 = Unbundle By Name(w444) -> ("nome collaudo"=w433:string, "QH regime.Curva 1"=w445:string[][], "QH regime.Curva 2"=w469:string[][], "QH regime.Curva 3"=w468:string[][])
              n120 = Index Array(array=w451, index=1) -> (element=w450:T6)
              n121 = Unbundle By Name(w460) -> ("QH"=w482:cluster{"X":dbl[], "Y":dbl[]}[], "QRPM"=w474:cluster{"X":dbl[], "Y":dbl[]}[], "QP2"=w467:cluster{"X":dbl[], "Y":dbl[]}[])
              n122 = Unbundle By Name(w450) -> ("Q"=w449:i32, "Htot"=w448:i32, "P2"=w447:i32)
              n123 = Multiply(x=w480, y=3) -> (x*y=w463:i32)
              n124 = call "GRAFICA CURVA XY.vi"("Y INDEX"=w448, "X INDEX"=w449, "Curva 1"=w445) -> ("Cluster"=w481:cluster{"X":dbl[], "Y":dbl[]})  [unwired: 8 in]
              n125 = call "GRAFICA CURVA XY.vi"("Y INDEX"=w448, "X INDEX"=w449, "Curva 1"=w469) -> ("Cluster"=w476:cluster{"X":dbl[], "Y":dbl[]})  [unwired: 8 in]
              n126 = call "GRAFICA CURVA XY.vi"("Y INDEX"=w448, "X INDEX"=w449, "Curva 1"=w468) -> ("Cluster"=w475:cluster{"X":dbl[], "Y":dbl[]})  [unwired: 8 in]
              n127 = call "GRAFICA CURVA XY.vi"("Y INDEX"=w471, "X INDEX"=w449, "Curva 1"=w445) -> ("Cluster"=w473:cluster{"X":dbl[], "Y":dbl[]})  [unwired: 8 in]
              n128 = call "GRAFICA CURVA XY.vi"("Y INDEX"=w471, "X INDEX"=w449, "Curva 1"=w469) -> ("Cluster"=w472:cluster{"X":dbl[], "Y":dbl[]})  [unwired: 8 in]
              n129 = call "GRAFICA CURVA XY.vi"("Y INDEX"=w471, "X INDEX"=w449, "Curva 1"=w468) -> ("Cluster"=w470:cluster{"X":dbl[], "Y":dbl[]})  [unwired: 8 in]
              n130 = call "GRAFICA CURVA XY.vi"("Y INDEX"=w447, "X INDEX"=w449, "Curva 1"=w445) -> ("Cluster"=w466:cluster{"X":dbl[], "Y":dbl[]})  [unwired: 8 in]
              n131 = call "GRAFICA CURVA XY.vi"("Y INDEX"=w447, "X INDEX"=w449, "Curva 1"=w469) -> ("Cluster"=w465:cluster{"X":dbl[], "Y":dbl[]})  [unwired: 8 in]
              n132 = call "GRAFICA CURVA XY.vi"("Y INDEX"=w447, "X INDEX"=w449, "Curva 1"=w468) -> ("Cluster"=w464:cluster{"X":dbl[], "Y":dbl[]})  [unwired: 8 in]
              n133 = Add(x=w463, y=2) -> (x+y=w461:i32)
              n134 = Add(x=w463, y=1) -> (x+y=w462:i32)
              n135 = Replace Array Subset(array=w482, new element #1=w481, index #1=w463, new element #2=w476, index #2=w462, new element #3=w475, index #3=w461) -> (w459:cluster{"X":dbl[], "Y":dbl[]}[])
              n136 = Replace Array Subset(array=w467, new element #1=w466, index #1=w463, new element #2=w465, index #2=w462, new element #3=w464, index #3=w461) -> (w457:cluster{"X":dbl[], "Y":dbl[]}[])
              n137 = Replace Array Subset(array=w474, new element #1=w473, index #1=w463, new element #2=w472, index #2=w462, new element #3=w470, index #3=w461) -> (w458:cluster{"X":dbl[], "Y":dbl[]}[])
              n138 = Unbundle By Name(w444) -> ("QH regime.Curva 1"=w443:string[][], "QH regime.Curva 2"=w442:string[][], "QH regime.Curva 3"=w441:string[][])
              n139 = Concatenate Strings(w433, "--Tab1" ("string")) -> (w456:string)
              n140 = Concatenate Strings(w433, "--Tab2" ("string")) -> (w455:string)
              n141 = Concatenate Strings(w433, "--Tab3" ("string")) -> (w454:string)
              n142 = Bundle By Name(cluster=w460, "QH"=w459, "QRPM"=w458, "QP2"=w457) -> (w453:T3)
              n143 = Build Array(w456, w455, w454) -> (w452:string[])
              n144 = Not Equal?(x=w440, y=w443) -> (x != y?=w438:bool)
              n145 = Not Equal?(x=w442, y=w440) -> (x != y?=w439:bool)
              n146 = Not Equal?(x=w441, y=w440) -> (x != y?=w437:bool)
              n147 = Build Array(w438, w439, w437) -> (w436:bool[])
            }
            frame "F" {
            }
            frame "T" {
            }
            frame "N" {
            }
          }
        }
        n148 = control-ref of="PLOT LEGEND QH-QRPM"() -> (w378:refnum<vi>)
        n149 = control-ref of="PLOT LEGEND QH-QH"() -> (w381:refnum<vi>)
        n150 = control-ref of="PLOT LEGEND QH-QP2"() -> (w380:refnum<vi>)
        n151 = local read "toll Q"() -> (w373:dbl)
        n152 = local read "toll H"() -> (w372:dbl)
        n153 = local read "Q2"() -> (w375:dbl)
        n154 = local read "H2"() -> (w374:dbl)
        n155 = local read "Q1"() -> (w377:dbl)
        n156 = local read "H1"() -> (w376:dbl)
        n157 = call "Croce.vi"("Solo toll Y positiva?"=FALSE, "TOLL Y %"=w372, "TOLL X %"=w373, "Grandezza Y"=w374, "grandezza X"=w375) -> ("element"=w368:cluster{"X":dbl[], "Y":dbl[]})  [unwired: 6 in]
        n158 = call "Croce.vi"("Solo toll Y positiva?"=FALSE, "TOLL Y %"=w372, "TOLL X %"=w373, "Grandezza Y"=w376, "grandezza X"=w377) -> ("element"=w369:cluster{"X":dbl[], "Y":dbl[]})  [unwired: 6 in]
        n159 = Build Array(w381, w378, w380) -> (w379:refnum<vi>[])
        n160 = Unbundle By Name(w366) -> ("QH"=w371:cluster{"X":dbl[], "Y":dbl[]}[])
        n161 = Array Size(array=w363) -> (size(s)=w358:i32)
        n162 = Increment(x=w358) -> (x+1=w370:i32)
        n163 = Replace Array Subset(array=w371, new element #1=w369, index #1=w358, new element #2=w368, index #2=w370) -> (w367:cluster{"X":dbl[], "Y":dbl[]}[])
        n164 = Build Array (concatenate)(w362, w365, w365) -> (w364:bool[])
        n165 = for {
          tunnel: w379 -> [w398] mode=indexing
          tunnel: w363 -> [w394]
          tunnel: w364 -> [w392]
          i -> [w395]
          n166 = case shown="2" w395 {
            tunnel: w394 -> [w403 w407 w413]
            tunnel: [w402 w407 w411] -> w393
            tunnel: w392 -> [w400 w406 w409]
            tunnel: [w399 w406 w408] -> w391
            frame 0, Default {
              w401 = TRUE
              n167 = Build Array (concatenate)(w403, "CROCE Q1H1", "CROCE Q2H2") -> (w402:string[])
              n168 = Build Array (concatenate)(w400, w401, w401) -> (w399:bool[])
            }
            frame 1 {
            }
            frame 2 {
              n169 = Build Array (concatenate)(w413, "CROCE Q2P2") -> (w411:string[])
              n170 = Build Array (concatenate)(w409, TRUE) -> (w408:bool[])
            }
          }
          n171 = property class="Arr (strict)"(reference=w398, "Value"=T2 []) -> (reference out=w396:refnum<vi>)  [unwired: 1 in, 1 out]
          n172 = for {
            shift-right: [w419] -> _
            shift-left: w396 -> [w421]
            tunnel: w393 -> [w416] mode=indexing
            tunnel: w391 -> [w414] mode=indexing
            i -> [w417]
            w415 = T11 {"nome plot"="Tab1\\18", "colore"=0, "Larghezza linea"=2, "stile linea"=0, "stile punto"=2, "Visibile?"=TRUE, "interpola?"=FALSE, "ordine"=2.0}  # valori default
            n173 = property class="Arr (strict)"(reference=w421) -> (reference out=w420:refnum<vi>, "Value"=w423:T2)  [unwired: 1 in, 1 out]
            n174 = Bundle By Name(cluster=w415, "nome plot"=w416, "Visibile?"=w414) -> (w418:T11)
            n175 = Insert Into Array(array=w423, index=w417, new element=w418) -> (w422:T2)
            n176 = property class="Arr (strict)"(reference=w420, "Value"=w422) -> (reference out=w419:refnum<vi>)  [unwired: 1 in, 1 out]
          }
        }
        n177 = local read "toll Q"() -> (w354:dbl)
        n178 = local read "toll P"() -> (w353:dbl)
        n179 = local read "Q2"() -> (w356:dbl)
        n180 = local read "P2"() -> (w355:dbl)
        n181 = Bundle By Name(cluster=w366, "QH"=w367) -> (w360:T3)
        n182 = call "Croce.vi"("Solo toll Y positiva?"=TRUE, "TOLL Y %"=w353, "TOLL X %"=w354, "Grandezza Y"=w355, "grandezza X"=w356) -> ("element"=w352:cluster{"X":dbl[], "Y":dbl[]})  [unwired: 6 in]
        n183 = Unbundle By Name(w360) -> ("QP2"=w359:cluster{"X":dbl[], "Y":dbl[]}[])
        n184 = Replace Array Subset(array=w359, new element=w352, index=w358) -> (w357:cluster{"X":dbl[], "Y":dbl[]}[])
        n185 = Bundle By Name(cluster=w360, "QP2"=w357) -> (w361:T3)
      }
      frame "Grafica" {
        n186 = Enqueue Element(queue=w485, element=cluster{"String":string, "variant":variant} {"String"="Grafica", "variant"=variant}) -> ()  [unwired: 2 in, 3 out]
        n187 = Wait (ms)(milliseconds to wait=u32 50) -> ()  [unwired: 1 out]
        n188 = control-ref of="PLOT LEGEND QH-QH"() -> (w490:refnum<vi>)
        n189 = control-ref of="PLOT LEGEND QH-QP2"() -> (w489:refnum<vi>)
        n190 = control-ref of="PLOT LEGEND QH-QRPM"() -> (w483:refnum<vi>)
        n191 = control-ref of="ProvaQH-QH"() -> (w492:refnum<vi>)
        n192 = control-ref of="ProvaQH-QRpm"() -> (w493:refnum<vi>)
        n193 = control-ref of="ProvaQH-QP2"() -> (w494:refnum<vi>)
        n194 = Unbundle By Name(w487) -> ("QH"=w498:cluster{"X":dbl[], "Y":dbl[]}[], "QRPM"=w497:cluster{"X":dbl[], "Y":dbl[]}[], "QP2"=w496:cluster{"X":dbl[], "Y":dbl[]}[])
        n195 = Build Array(w498, w497, w496) -> (w495:cluster{"X":dbl[], "Y":dbl[]}[][])
        n196 = Build Array(w492, w493, w494) -> (w491:refnum<vi>[])
        n197 = Build Array(w490, w483, w489) -> (w488:refnum<vi>[])
        n198 = for {
          tunnel: w491 -> [w504] mode=indexing
          tunnel: w495 -> [w503] mode=indexing
          tunnel: w488 -> [w502] mode=indexing
          n199 = call "Gestione grafico.vi"("graph ref"=w504, "PLOT LEGEND"=w502, "Array"=w503) -> ("Array out"=w505:cluster{"X":dbl[], "Y":dbl[]}[])  [unwired: 8 in]
          n200 = property class="XYGraph (strict)"(reference=w504, "Value"=w505) -> ()  [unwired: 1 in, 2 out]
        }
      }
      frame "REPORT EXCEL" {
        n201 = stacked-sequence {
          seq-local: [w513 _ _] -> [_ _ w580]
          seq-local: [w512 _ _] -> [_ _ w576]
          seq-local: [w511 _ _] -> [_ _ w571]
          tunnel: w507 -> [_ _ w564]
          tunnel: w506 -> [_ _ w553]
          frame #0 {
            w514 = 70 ("quality (80)")
            n202 = control-ref of="ProvaQH-QP2"() -> (w515:refnum<vi>)
            n203 = control-ref of="ProvaQH-QRpm"() -> (w525:refnum<vi>)
            n204 = control-ref of="ProvaQH-QH"() -> (w510:refnum<vi>)
            n205 = call <vilib>:"Application Directory.vi"() -> ("Application Directory"=w530:path)
            n206 = call <vilib>:"Application Directory.vi"() -> ("Application Directory"=w523:path)
            n207 = call <vilib>:"Application Directory.vi"() -> ("Application Directory"=w516:path)
            n208 = invoke class="XYGraph (strict)" method="Get Image"(reference=w525, "bg color"=u32 16448250) -> ("image data"=w524:T12)  [unwired: 4 in, 5 out]
            n209 = invoke class="XYGraph (strict)" method="Get Image"(reference=w515, "bg color"=u32 16448250) -> ("image data"=w518:T12)  [unwired: 4 in, 5 out]
            n210 = invoke class="XYGraph (strict)" method="Get Image"(reference=w510, "bg color"=u32 16448250) -> ("image data"=w531:T12)  [unwired: 4 in, 5 out]
            n211 = Build Path(base path=w530, name or relative path="Report\\Immagini temp\\QH_QH.jpeg") -> (appended path=w528:path)
            n212 = Build Path(base path=w523, name or relative path="Report\\Immagini temp\\QH_QRpm.jpeg") -> (appended path=w522:path)
            n213 = Build Path(base path=w516, name or relative path="Report\\Immagini temp\\QH_QP2.jpeg") -> (appended path=w519:path)
            n214 = call <vilib>:"Write JPEG File.vi"("quality (80)"=w514, "image data"=w531, "path to JPEG file"=w528) -> ("path"=w513:path)  [unwired: 7 in, 1 out]
            n215 = call <vilib>:"Write JPEG File.vi"("quality (80)"=w514, "image data"=w524, "path to JPEG file"=w522) -> ("path"=w512:path)  [unwired: 7 in, 1 out]
            n216 = call <vilib>:"Write JPEG File.vi"("quality (80)"=w514, "image data"=w518, "path to JPEG file"=w519) -> ("path"=w511:path)  [unwired: 7 in, 1 out]
          }
          frame #1 {
            n217 = Wait (ms)(milliseconds to wait=u32 2000) -> ()  [unwired: 1 out]
          }
          frame #2 {
            w535 = enum16{"Virgola", "Punto"}."Punto"  # sep. decimale numeri esportati
            n218 = Unbundle By Name(w564) -> ("QH regime.Curva 1"=w563:string[][], "QH regime.Curva 2"=w561:string[][], "QH regime.Curva 3"=w560:string[][])
            n219 = local read "Nomi colonne"() -> (w562:string[])
            n220 = Build Array (concatenate)(w562, w563) -> (w539:string[][])
            n221 = Build Array (concatenate)(w562, w561) -> (w537:string[][])
            n222 = Build Array (concatenate)(w562, w560) -> (w534:string[][])
            n223 = call <vilib>:"New Report.vi"("window state (normal)"=T4."no change", "report type"=T5."Excel", "template (empty)"="template (empty) 2") -> ("report out"=w557:refnum<class "NI_report.lvclass">, "error out"=w558:errorcluster)  [unwired: 11 in]
            n224 = case shown="\"Punto\"" w535 {
              tunnel: w539 -> [w618 w626]
              tunnel: [w617 w625] -> w538
              frame "Virgola", Default {
                n225 = for {
                  tunnel: w618 -> [w620] mode=indexing
                  tunnel: [w619] -> w617 mode=indexing
                  n226 = for {
                    tunnel: w620 -> [w624] mode=indexing
                    tunnel: [w621] -> w619 mode=indexing
                    n227 = Search and Replace String(input string=w624, search string=",", replace string="." ("search string")) -> (result string=w621:string)  [unwired: 5 in, 3 out]
                  }
                }
              }
              frame "Punto" {
                n228 = for {
                  tunnel: w626 -> [w628] mode=indexing
                  tunnel: [w627] -> w625 mode=indexing
                  n229 = for {
                    tunnel: w628 -> [w632] mode=indexing
                    tunnel: [w629] -> w627 mode=indexing
                    n230 = Search and Replace String(input string=w632, search string=".", replace string="," ("search string")) -> (result string=w629:string)  [unwired: 5 in, 3 out]
                  }
                }
              }
            }
            n231 = case shown="\"Punto\"" w535 {
              tunnel: w537 -> [w602 w610]
              tunnel: [w601 w609] -> w536
              frame "Virgola", Default {
                n232 = for {
                  tunnel: w602 -> [w604] mode=indexing
                  tunnel: [w603] -> w601 mode=indexing
                  n233 = for {
                    tunnel: w604 -> [w608] mode=indexing
                    tunnel: [w605] -> w603 mode=indexing
                    n234 = Search and Replace String(input string=w608, search string=",", replace string="." ("search string")) -> (result string=w605:string)  [unwired: 5 in, 3 out]
                  }
                }
              }
              frame "Punto" {
                n235 = for {
                  tunnel: w610 -> [w612] mode=indexing
                  tunnel: [w611] -> w609 mode=indexing
                  n236 = for {
                    tunnel: w612 -> [w616] mode=indexing
                    tunnel: [w613] -> w611 mode=indexing
                    n237 = Search and Replace String(input string=w616, search string=".", replace string="," ("search string")) -> (result string=w613:string)  [unwired: 5 in, 3 out]
                  }
                }
              }
            }
            n238 = case shown="\"Punto\"" w535 {
              tunnel: w534 -> [w586 w594]
              tunnel: [w585 w593] -> w533
              frame "Virgola", Default {
                n239 = for {
                  tunnel: w586 -> [w588] mode=indexing
                  tunnel: [w587] -> w585 mode=indexing
                  n240 = for {
                    tunnel: w588 -> [w592] mode=indexing
                    tunnel: [w589] -> w587 mode=indexing
                    n241 = Search and Replace String(input string=w592, search string=",", replace string="." ("search string")) -> (result string=w589:string)  [unwired: 5 in, 3 out]
                  }
                }
              }
              frame "Punto" {
                n242 = for {
                  tunnel: w594 -> [w596] mode=indexing
                  tunnel: [w595] -> w593 mode=indexing
                  n243 = for {
                    tunnel: w596 -> [w600] mode=indexing
                    tunnel: [w597] -> w595 mode=indexing
                    n244 = Search and Replace String(input string=w600, search string=".", replace string="," ("search string")) -> (result string=w597:string)  [unwired: 5 in, 3 out]
                  }
                }
              }
            }
            n245 = call <vilib>:"Excel Get Worksheet.vi"("report in"=w557, "error in (no error)"=w558, "name (\"\")"="Dati_nascosti" ("name (\"\")")) -> ("report out"=w555:refnum<class "NI_report.lvclass">, "error out"=w554:errorcluster)  [unwired: 11 in]
            n246 = call-poly <vilib>:"Excel Easy Table.vi"("report in"=w555, "text data"=w553, "error in (no error)"=w554) -> ("report out"=w551:refnum<class "NI_report.lvclass">, "error out"=w550:errorcluster)  [unwired: 8 in, 3 out]
            n247 = call-poly <vilib>:"Excel Easy Table.vi"("report in"=w551, "start (0, 0)"=cluster{"row":i32, "column":i32} {"row"=5, "column"=0}, "text data"=w538, "error in (no error)"=w550) -> ("report out"=w548:refnum<class "NI_report.lvclass">, "error out"=w549:errorcluster)  [unwired: 7 in, 3 out]
            n248 = call-poly <vilib>:"Excel Easy Table.vi"("report in"=w548, "start (0, 0)"=cluster{"row":i32, "column":i32} {"row"=55, "column"=0}, "text data"=w536, "error in (no error)"=w549) -> ("report out"=w545:refnum<class "NI_report.lvclass">, "error out"=w546:errorcluster)  [unwired: 7 in, 3 out]
            n249 = call-poly <vilib>:"Excel Easy Table.vi"("report in"=w545, "start (0, 0)"=cluster{"row":i32, "column":i32} {"row"=105, "column"=0}, "text data"=w533, "error in (no error)"=w546) -> ("report out"=w543:refnum<class "NI_report.lvclass">, "error out"=w542:errorcluster)  [unwired: 7 in, 3 out]
            n250 = call <vilib>:"Excel Get Worksheet.vi"("report in"=w543, "error in (no error)"=w542, "name (\"\")"="grafici" ("name (\"\")")) -> ("report out"=w581:refnum<class "NI_report.lvclass">, "error out"=w582:errorcluster)  [unwired: 11 in]
            n251 = call-poly <vilib>:"Append Image to Report.vi"("report in"=w581, "MS Office parameters"=T7 {"position (Excel)"={"row"=19, "column"=0}, "name (Excel)"="", "bookmark (Word)"=""}, "path or URL of image"=w580, "error in (no error)"=w582) -> ("report out"=w578:refnum<class "NI_report.lvclass">, "error out"=w577:errorcluster)  [unwired: 8 in, 2 out]
            n252 = call "File Dialog"("pattern (all files)"=".xls") -> ("selected path"=w567:path)  [unwired: 11 in, 3 out]
            n253 = call-poly <vilib>:"Append Image to Report.vi"("report in"=w578, "MS Office parameters"=T7 {"position (Excel)"={"row"=47, "column"=0}, "name (Excel)"="", "bookmark (Word)"=""}, "path or URL of image"=w576, "error in (no error)"=w577) -> ("report out"=w573:refnum<class "NI_report.lvclass">, "error out"=w574:errorcluster)  [unwired: 8 in, 2 out]
            n254 = call-poly <vilib>:"Append Image to Report.vi"("report in"=w573, "MS Office parameters"=T7 {"position (Excel)"={"row"=66, "column"=0}, "name (Excel)"="", "bookmark (Word)"=""}, "path or URL of image"=w571, "error in (no error)"=w574) -> ("report out"=w569:refnum<class "NI_report.lvclass">, "error out"=w570:errorcluster)  [unwired: 8 in, 2 out]
            n255 = call-dynamic "Save Report to File.vi"("report in"=w569, "report file path"=w567, "prompt to replace? (F)"=TRUE, "error in (no error)"=w570) -> ("report out"=w540:refnum<class "NI_report.lvclass">, "error out"=w541:errorcluster)  [unwired: 10 in]
            n256 = call-dynamic "Dispose Report.vi"("report in"=w540, "error in (no error)"=w541) -> ()  [unwired: 13 in, 1 out]
          }
        }
      }
      frame "exit" {
      }
    }
  }
  n257 = disable-structure shown="Disabled" {
    frame Disabled {
    }
    frame Enabled {
    }
  }
